vi "time.vi"(0 "buffer in":string) -> (1 "mm:ss":string, 2 "minutes":dbl, 3 "seconds":dbl)   [LabVIEW 2016]
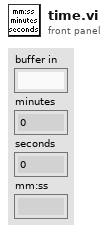
[diagram p1: front panel]
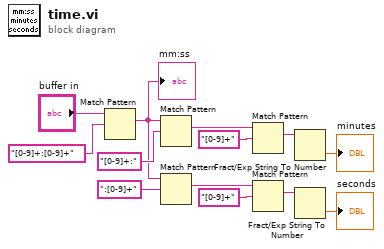
[diagram p0: block diagram]
diagram:
  n1 = Match Pattern(string="buffer in", regular expression="[0-9]+:[0-9]+") -> (match substring=w1:string)  [unwired: 1 in, 3 out]
  "mm:ss" <- w1
  n2 = Match Pattern(string=w1, regular expression="[0-9]+:") -> (match substring=w9:string)  [unwired: 1 in, 3 out]
  n3 = Match Pattern(string=w1, regular expression=":[0-9]+") -> (match substring=w4:string)  [unwired: 1 in, 3 out]
  n4 = Match Pattern(string=w9, regular expression="[0-9]+") -> (match substring=w8:string)  [unwired: 1 in, 3 out]
  n5 = Match Pattern(string=w4, regular expression="[0-9]+") -> (match substring=w3:string)  [unwired: 1 in, 3 out]
  n6 = Fract/Exp String To Number(string=w8) -> (number=→"minutes":dbl)  [unwired: 3 in, 1 out]
  n7 = Fract/Exp String To Number(string=w3) -> (number=→"seconds":dbl)  [unwired: 3 in, 1 out]
